vi "全局 1.vi"() -> ()   [LabVIEW 2017]
panel:
  in  "音频播放索引":i32[](array[numeric])
  in  "database路径":path=path "D:/桌面文件/1aatest/主控"
  in  "主程序路径":path=path "D:/桌面文件/1aatest/主控"
  in  "退出":bool
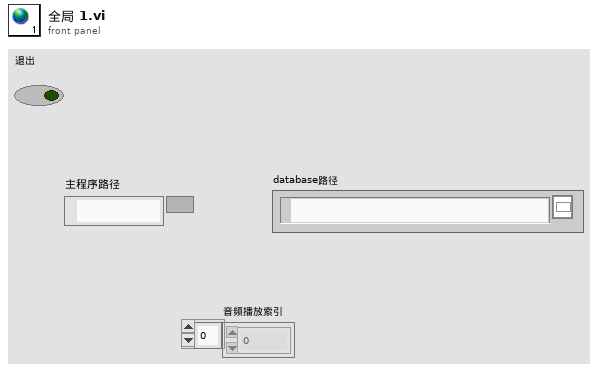
[diagram p1: front panel]
diagram:
